vi "Main.vi"(10 "VISA resource name":refnum<visa-resource-name>, 11 "Module Admin":refnum<class "Delacor_lib_QMH_Cloneable Module Admin.lvclass">) -> ()   [LabVIEW 2018, in "CE14_v3.lvlib"]
doc: "This template is based off of the Queued Message Handler design pattern and the Queued Message Handler project template that ships with LabVIEW.\n\nThe main difference is that the queue is private to this module and communication between modules is performed via Broadcast and Request events.\n\nRequest events are wrapped in public API methods and are handled in the Event Handling Loop (EHL) of this VI. Any module can register for Broadcast events sent by this module. The EHL generates messages based on user interface actions.\n\nThe Message Handling Loop (MHL) processes messages generated by the EHL, or by other messages. The messages are string values, so new messages can be added easily to the Message Cases case structure in the MHL. Each message cluster can also provide an optional value for Message Data, which is a variant that can be converted to whatever message-specific data is required.\n_____\nBased on DQMH Project Template 6.0.0.91."
uses:
  CE14_v3.lvlib
  <vilib>/Delacor/Delacor QMH/Libraries/Cloneable Module Admin_class/Delacor_lib_QMH_Cloneable Module Admin.lvclass
  C:/Program Files (x86)/National Instruments/LabVIEW 2018/vi.lib/Delacor/Delacor QMH/Libraries/Module Admin_class/Delacor_lib_QMH_Module Admin.lvclass
  Module Data--cluster.ctl
  <vilib>/Delacor/Delacor QMH/Libraries/Message Queue_class/Delacor_lib_QMH_Message Queue.lvclass/Delacor_lib_QMH_Message Queue.ctl
  <vilib>/Delacor/Delacor QMH/Libraries/Cloneable Module Admin_class/Delacor_lib_QMH_Cloneable Module Admin.lvclass/Delacor_lib_QMH_Cloneable Module Admin.ctl
  Stop Argument--cluster.ctl
  <vilib>/Delacor/Delacor QMH/Libraries/Module Admin_class/Delacor_lib_QMH_Module Admin.lvclass/Delacor_lib_QMH_Module Admin.ctl
  CE14 Open and Shakehand Argument--cluster.ctl
  Check Shakehand Success Argument--cluster.ctl
  Check Shakehand Success (Reply Payload)--cluster.ctl
  <vilib>/Utility/miscctls.llb/LVPointTypeDef.ctl
  <vilib>/Delacor/Delacor QMH/Libraries/Message Queue_class/Delacor_lib_QMH_Enqueue Message (Single).vi
  <vilib>/Delacor/Delacor QMH/Libraries/Cloneable Module Admin_class/Delacor_lib_QMH_Get Module ID.vi
  <vilib>/Delacor/Delacor QMH/Libraries/Module Admin_class/Delacor_lib_QMH_Get External Launch.vi
  <vilib>/Utility/error.llb/Error Cluster From Error Code.vi
  <vilib>/ErrorRing/Error Ring.xnode
  <vilib>/Delacor/Delacor QMH/Libraries/Message Queue_class/Delacor_lib_QMH_Message Queue.lvclass
  Instrument Drivers/LVdriver_CE14(eMIC)/CE14_eMIC.lvlib
panel:
  out "error out":errorcluster
  out "Status":string
  in  "Simulate EHL Error":bool
  in  "Simulate MHL Error":bool
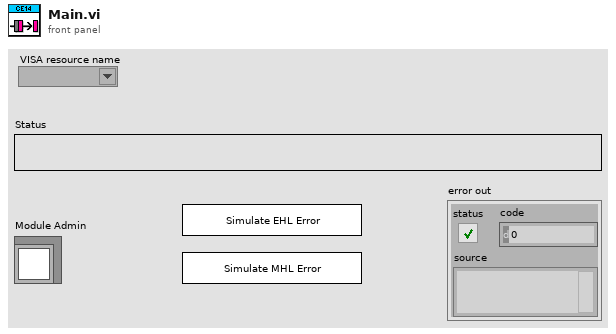
[diagram p1: front panel]
types:
  T1 = typedef "CE14_v3.lvlib/Request Events--cluster.ctl" = cluster{"Stop Module":refnum<user-event>, "Show Panel":refnum<user-event>, "Hide Panel":refnum<user-event>, "Show Diagram":refnum<user-event>, "Get Module Execution Status":refnum<user-event>, "CE14 Open and Shakehand":refnum<user-event>, "Check Shakehand Success":refnum<user-event>}
  T2 = typedef "CE14_v3.lvlib/Module Data--cluster.ctl" = cluster{"Status":string, "VISA resource name":refnum<visa-resource-name>, "ShakeHand Success?":bool}
  T3 = enum32{"invalid lock state", "Not Locked", "Locked (No Password)", "Password-protected"}
  T4 = typedef "CE14_v3.lvlib/Stop Argument--cluster.ctl" = cluster{"Module ID":i32, "Origin":string, "Exit via Stop Module Req?":bool, "Wait for Module to stop?":bool}
  T5 = typedef "CE14_v3.lvlib/CE14 Open and Shakehand Argument--cluster.ctl" = cluster{"Module ID":i32, "Boolean":bool}
  T6 = typedef "CE14_v3.lvlib/Check Shakehand Success Argument--cluster.ctl" = cluster{"Module ID":i32, "Wait Notifier":refnum<notifier>, "wait for reply":bool}
  T7 = typedef "LVPointTypeDef.ctl" = cluster{"Horizontal":i16, "Vertical":i16}
  T8 = enum32{"Invalid", "Standard", "Closed", "Hidden", "Minimized", "Maximized"}
  T9 = typedef "CE14_v3.lvlib/Check Shakehand Success (Reply Payload)--cluster.ctl" = cluster{"ShakeHand Success?":bool, "Check Shakehand Success_error":errorcluster}
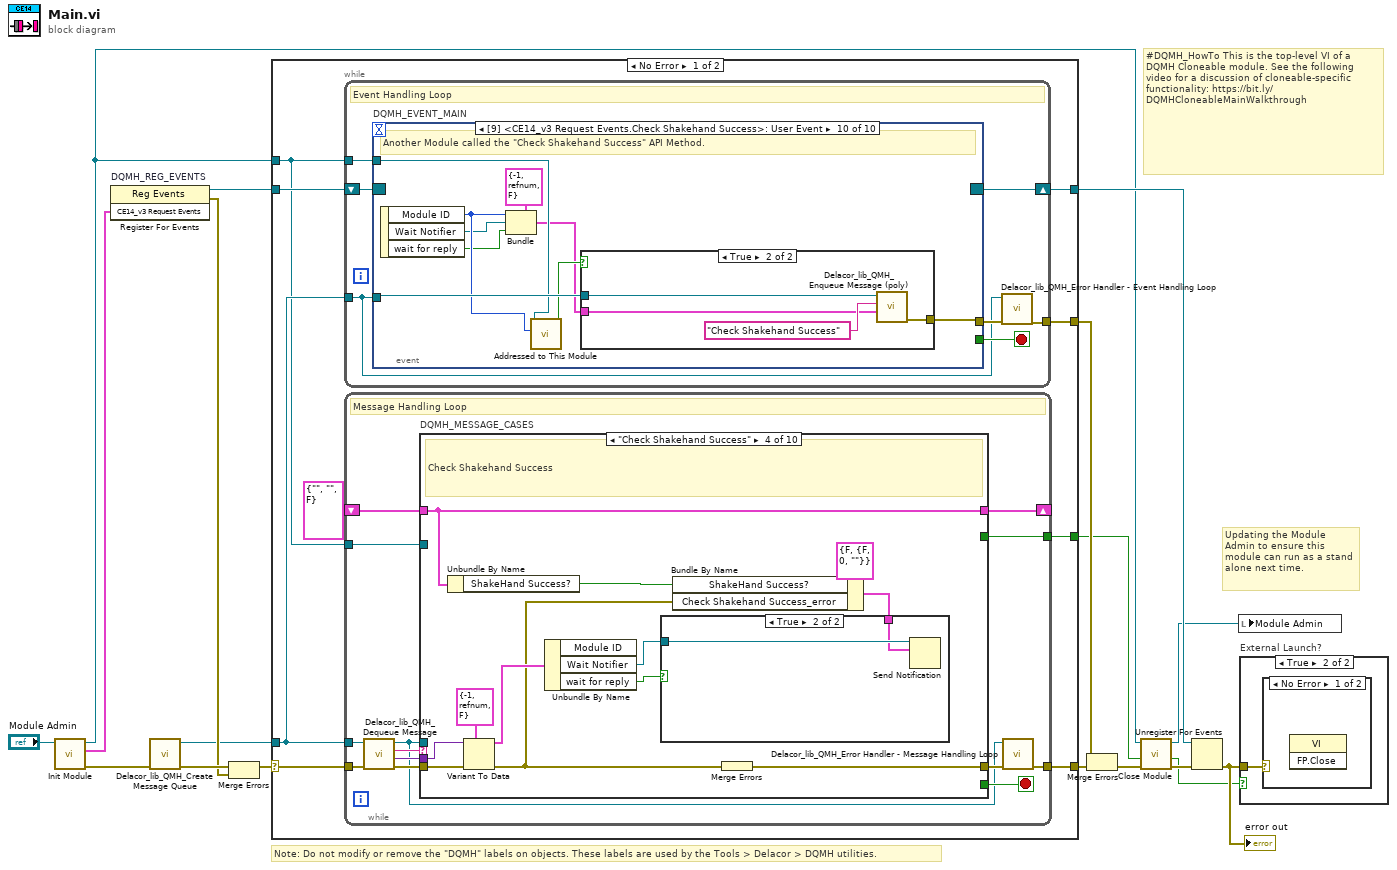
[diagram p0: block diagram]
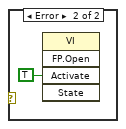
[diagram p3: hidden frame]
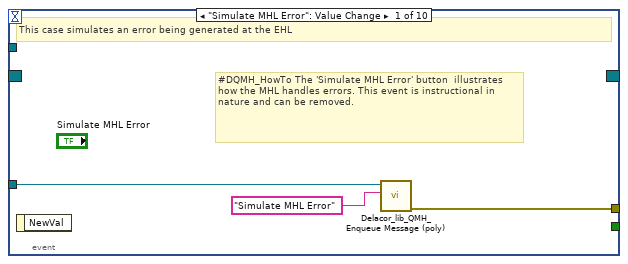
[diagram p4: hidden frame]
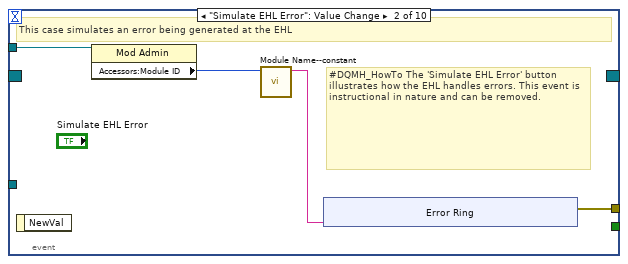
[diagram p5: hidden frame]
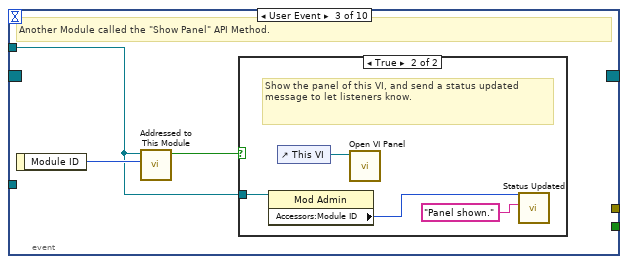
[diagram p6: hidden frame]
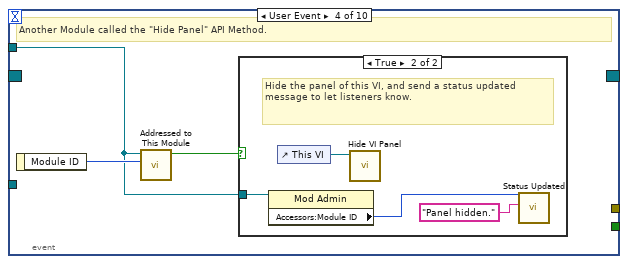
[diagram p8: hidden frame]
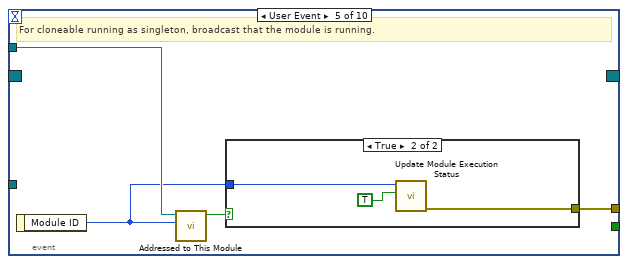
[diagram p10: hidden frame]
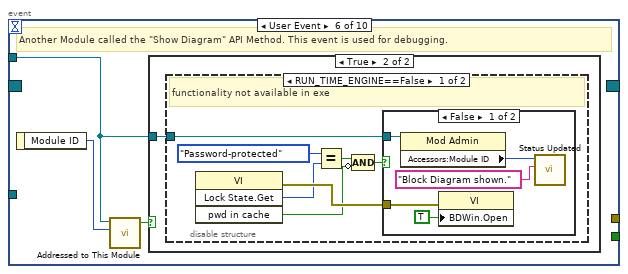
[diagram p12: hidden frame]
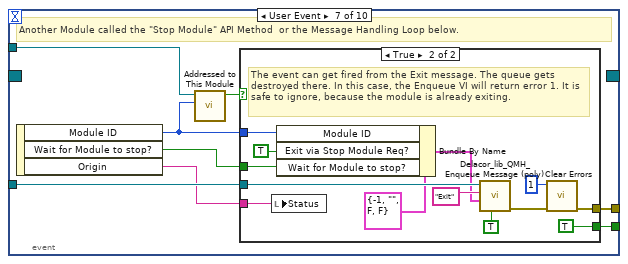
[diagram p16: hidden frame]
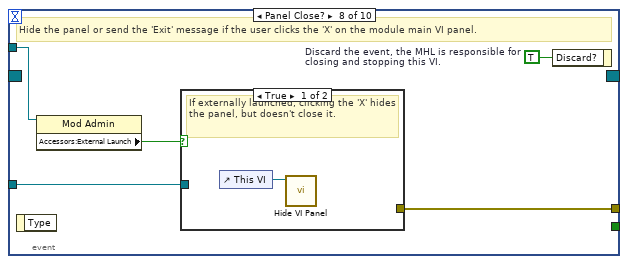
[diagram p18: hidden frame]
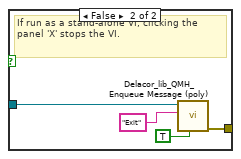
[diagram p19: hidden frame]
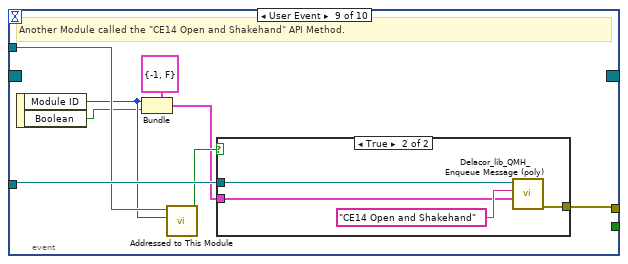
[diagram p20: hidden frame]
diagram:
  # "#DQMH_HowTo This is the top-level VI of a DQMH Cloneable module. See the following video for a discussion of cloneable-specific functionality: https://bit.ly/DQMHCloneableMainWalkthrough"
  # "Note: Do not modify or remove the \"DQMH\" labels on objects. These labels are used by the Tools > Delacor > DQMH utilities."
  # "Updating the Module Admin to ensure this module can run as a stand alone next time."
  n1 = call "Init Module.vi"("Cloneable Module Admin in"="Module Admin") -> ("error out"=w15:errorcluster, "CE14_v3 Request Events"=w7:T1, "Cloneable Module Admin out"=w4:refnum<class "Delacor_lib_QMH_Cloneable Module Admin.lvclass">)  [unwired: 8 in]
  n2 = register-events "DQMH_REG_EVENTS"(w7) -> (reference out=w8:refnum<event-registration>, error out=w10:errorcluster)  [unwired: 2 in]
  n3 = call <vilib>:"Delacor_lib_QMH_Create Message Queue.vi"("error in"=w15) -> ("error out"=w12:errorcluster, "Message Queue"=w6:refnum<class "Delacor_lib_QMH_Message Queue.lvclass">)  [unwired: 9 in]
  n4 = Merge Errors(w12, w10) -> (w11:errorcluster)
  n5 = case shown="No Error" w11 {
    selector: w11 -> [w25 w274]
    tunnel: [w27 w273] -> w16
    tunnel: [w24 w281] -> w9
    tunnel: w8 -> [w22 w281]
    tunnel: w6 -> [w21 w272]
    tunnel: [w26 _] -> w17
    tunnel: w4 -> [w20 w277]
    tunnel: [w19 _] -> w2
    frame No Error {
      n6 = while {
        tunnel: w21 -> [w28]
        shift-right: [w31] -> w24
        shift-left: w22 -> [w32]
        tunnel: [w33] -> w26
        tunnel: w20 -> [w29]
        stop <- w30 stop-if-true
        # "Event Handling Loop"
        n7 = event "DQMH_EVENT_MAIN" shown="[9] <CE14_v3 Request Events.Check Shakehand Success>: User Event" {
          selector: w32 -> [_ _ _ _ _ _ _ _ _ _]
          dyn-events: [_ _ _ _ _ _ _ _ _ _] -> w31
          timeout: _ -> [_ _ _ _ _ _ _ _ _ _]
          tunnel: [_ _ _ _ _ _ w89 _ _ _] -> w30
          tunnel: w28 -> [w36 _ _ _ _ _ w92 w108 w124 w137]
          tunnel: [w37 w41 _ _ w66 _ w93 w111 w117 w129] -> w34
          tunnel: w29 -> [_ w40 w49 w56 w64 w70 w91 w109 w122 w135]
          event "Simulate MHL Error": Value Change {
            # "#DQMH_HowTo The 'Simulate MHL Error' button  illustrates how the MHL handles errors. This event is instructional in nature and can be removed."
            # "This case simulates an error being generated at the EHL"
            n8 = event-data() -> ()  [unwired: 1 in, 1 out]
            n9 = call-poly <vilib>:"Delacor_lib_QMH_Enqueue Message (poly).vi"("Message"="Simulate MHL Error", "Message Queue in"=w36) -> ("error out"=w37:errorcluster)  [unwired: 8 in, 1 out]
          }
          event "Simulate EHL Error": Value Change {
            # "#DQMH_HowTo The 'Simulate EHL Error' button  illustrates how the EHL handles errors. This event is instructional in nature and can be removed."
            # "This case simulates an error being generated at the EHL"
            n10 = event-data() -> ()  [unwired: 1 in, 1 out]
            n11 = property class="Mod Admin"(reference=w40) -> ("Accessors:Module ID"=w39:i32)  [unwired: 1 in, 2 out]
            n12 = call "Module Name--constant.vi"("Module ID"=w39) -> ("Module Name"=w38:string)  [unwired: 10 in]
            n13 = xnode "Error Ring"("parameter 0"=w38) -> ("error out"=w41:errorcluster)
          }
          event User Event {
            # "Another Module called the \"Show Panel\" API Method."
            n14 = event-data() -> ("Module ID"=w50:i32)  [unwired: 1 in]
            n15 = call "Addressed to This Module.vi"("Module ID from Argument"=w50, "Module Admin"=w49) -> ("Addressed to this instance?"=w51:bool)  [unwired: 8 in, 1 out]
            n16 = case shown="True" w51 {
              tunnel: w49 -> [_ w53]
              frame False {
              }
              frame True {
                # "Show the panel of this VI, and send a status updated message to let listeners know."
                n17 = property class="Mod Admin"(reference=w53) -> ("Accessors:Module ID"=w52:i32)  [unwired: 1 in, 2 out]
                n18 = control-ref of="This VI"() -> (w55:refnum<vi>)
                n19 = call "Open VI Panel.vi"("VI"=w55) -> ()  [unwired: 10 in, 1 out]
                n20 = call "Status Updated.vi"("Status"="Panel shown." ("format string"), "Module ID"=w52) -> ()  [unwired: 9 in, 1 out]
              }
            }
          }
          event User Event {
            # "Another Module called the \"Hide Panel\" API Method."
            n21 = event-data() -> ("Module ID"=w57:i32)  [unwired: 1 in]
            n22 = call "Addressed to This Module.vi"("Module ID from Argument"=w57, "Module Admin"=w56) -> ("Addressed to this instance?"=w58:bool)  [unwired: 8 in, 1 out]
            n23 = case shown="True" w58 {
              tunnel: w56 -> [_ w60]
              frame False {
              }
              frame True {
                # "Hide the panel of this VI, and send a status updated message to let listeners know."
                n24 = property class="Mod Admin"(reference=w60) -> ("Accessors:Module ID"=w59:i32)  [unwired: 1 in, 2 out]
                n25 = control-ref of="This VI"() -> (w62:refnum<vi>)
                n26 = call "Hide VI Panel.vi"("VI"=w62) -> ()  [unwired: 10 in, 1 out]
                n27 = call "Status Updated.vi"("Status"="Panel hidden." ("format string"), "Module ID"=w59) -> ()  [unwired: 9 in, 1 out]
              }
            }
          }
          event User Event {
            # "For cloneable running as singleton, broadcast that the module is running."
            n28 = event-data() -> ("Module ID"=w63:i32)  [unwired: 1 in]
            n29 = call "Addressed to This Module.vi"("Module ID from Argument"=w63, "Module Admin"=w64) -> ("Addressed to this instance?"=w65:bool)  [unwired: 8 in, 1 out]
            n30 = case shown="True" w65 {
              tunnel: [_ w69] -> w66
              tunnel: w63 -> [_ w68]
              frame False {
              }
              frame True {
                n31 = call "Update Module Execution Status.vi"("Running?"=TRUE, "Module ID"=w68) -> ("error out"=w69:errorcluster)  [unwired: 9 in]
              }
            }
          }
          event User Event {
            # "Another Module called the \"Show Diagram\" API Method. This event is used for debugging."
            n32 = event-data() -> ("Module ID"=w71:i32)  [unwired: 1 in]
            n33 = call "Addressed to This Module.vi"("Module ID from Argument"=w71, "Module Admin"=w70) -> ("Addressed to this instance?"=w72:bool)  [unwired: 8 in, 1 out]
            n34 = case shown="True" w72 {
              tunnel: w70 -> [_ w73]
              frame False {
              }
              frame True {
                n35 = disable-structure shown="RUN_TIME_ENGINE==False" {
                  disable-tunnel: w73 -> [w74 _]
                  frame condition #0 (active) {
                    # "functionality not available in exe"
                    n36 = invoke class="VI" method="Lock State.Get"() -> (error out=w80:errorcluster, "Get Lock State"=w79:T3, "pwd in cache"=w76:bool)  [unwired: 4 in, 1 out]
                    n37 = Equal?(x=T3."Password-protected", y=w79) -> (x = y?=w77:bool)
                    n38 = Compound Arithmetic op=AND(w77, invert w76) -> (w75:bool)
                    n39 = case shown="False" w75 {
                      tunnel: w80 -> [w85 _]
                      tunnel: w74 -> [w82 _]
                      frame False {
                        n40 = property class="Mod Admin"(reference=w82) -> ("Accessors:Module ID"=w81:i32)  [unwired: 1 in, 2 out]
                        n41 = property class="VI"(error in=w85, "BDWin.Open"=TRUE ("Block Diagram Window:Open")) -> ()  [unwired: 1 in, 2 out]
                        n42 = call "Status Updated.vi"("Status"="Block Diagram shown." ("format string"), "Module ID"=w81) -> ()  [unwired: 9 in, 1 out]
                      }
                      frame True {
                        # "Password-protected VI, and the password is not in the cache. Do not show the diagram."
                      }
                    }
                  }
                  frame condition #1 {
                  }
                }
              }
            }
          }
          event User Event {
            # "Another Module called the \"Stop Module\" API Method  or the Message Handling Loop below."
            n43 = event-data() -> ("Module ID"=w87:i32, "Wait for Module to stop?"=w88:bool, "Origin"=w86:string)  [unwired: 1 in]
            n44 = call "Addressed to This Module.vi"("Module ID from Argument"=w87, "Module Admin"=w91) -> ("Addressed to this instance?"=w90:bool)  [unwired: 8 in, 1 out]
            n45 = case shown="True" w90 {
              tunnel: [_ w105] -> w93
              tunnel: w92 -> [_ w101]
              tunnel: [_ TRUE] -> w89
              tunnel: w88 -> [_ w96]
              tunnel: w87 -> [_ w98]
              tunnel: w86 -> [_ w94]
              frame False {
              }
              frame True {
                # "The event can get fired from the Exit message. The queue gets destroyed there. In this case, the Enqueue VI will return error 1. It is safe to ignore, because the module is already exiting."
                n46 = local write "Status"(w94) -> ()
                n47 = Bundle By Name(cluster=T4 {"Module ID"=-1, "Origin"="", "Exit via Stop Module Req?"=FALSE, "Wait for Module to stop?"=FALSE} ("Stop Argument"), "Module ID"=w98, "Exit via Stop Module Req?"=TRUE, "Wait for Module to stop?"=w96) -> (w95:T4)
                n48 = call-poly <vilib>:"Delacor_lib_QMH_Enqueue Message (poly).vi"("Priority Message? (F)"=TRUE, "Message Data"=w95, "Message"="Exit", "Message Queue in"=w101) -> ("error out"=w106:errorcluster)  [unwired: 6 in, 1 out]
                n49 = call <vilib>:"Clear Errors.vi"("error in (no error)"=w106, "specific error code to clear (0: all)"=1) -> ("error out"=w105:errorcluster)  [unwired: 4 in, 1 out]
              }
            }
          }
          event Panel Close? {
            w110 = TRUE  # Discard the event, the MHL is responsible for closing and stopping this VI.
            # "Hide the panel or send the 'Exit' message if the user clicks the 'X' on the module main VI panel."
            n50 = event-data() -> ()  [unwired: 1 in, 1 out]
            n51 = property class="Mod Admin"(reference=w109) -> ("Accessors:External Launch"=w107:bool)  [unwired: 1 in, 2 out]
            n52 = case shown="True" w107 {
              tunnel: w108 -> [_ w115]
              tunnel: [_ w116] -> w111
              frame True {
                # "If externally launched, clicking the 'X' hides the panel, but doesn't close it."
                n53 = control-ref of="This VI"() -> (w112:refnum<vi>)
                n54 = call "Hide VI Panel.vi"("VI"=w112) -> ()  [unwired: 10 in, 1 out]
              }
              frame False {
                # "If run as a stand-alone VI, clicking the panel 'X' stops the VI."
                n55 = call-poly <vilib>:"Delacor_lib_QMH_Enqueue Message (poly).vi"("Priority Message? (F)"=TRUE, "Message"="Exit", "Message Queue in"=w115) -> ("error out"=w116:errorcluster)  [unwired: 7 in, 1 out]
              }
            }
            n56 = event-data("Discard?"=w110) -> ()  [unwired: 1 in, 1 out]
          }
          event User Event {
            # "Another Module called the \"CE14 Open and Shakehand\" API Method."
            n57 = event-data() -> ("Module ID"=w119:i32, "Boolean"=w118:bool)  [unwired: 1 in]
            n58 = Bundle(cluster=T5 {"Module ID"=-1, "Boolean"=FALSE} ("CE14 Open and Shakehand Argument"), "Module ID"=w119, "Boolean"=w118) -> (w120:T5)
            n59 = call "Addressed to This Module.vi"("Module ID from Argument"=w119, "Module Admin"=w122) -> ("Addressed to this instance?"=w123:bool)  [unwired: 8 in, 1 out]
            n60 = case shown="True" w123 {
              tunnel: w124 -> [_ w128]
              tunnel: w120 -> [_ w126]
              tunnel: [_ w125] -> w117
              frame False {
              }
              frame True {
                n61 = call-poly <vilib>:"Delacor_lib_QMH_Enqueue Message (poly).vi"("Message Data"=w126, "Message"="CE14 Open and Shakehand", "Message Queue in"=w128) -> ("error out"=w125:errorcluster)  [unwired: 7 in, 1 out]
              }
            }
          }
          event User Event {
            # "Another Module called the \"Check Shakehand Success\" API Method."
            n62 = event-data() -> ("Module ID"=w132:i32, "Wait Notifier"=w131:refnum<notifier>, "wait for reply"=w130:bool)  [unwired: 1 in]
            n63 = Bundle(cluster=T6 {"Module ID"=-1, "Wait Notifier"=refnum, "wait for reply"=FALSE} ("Check Shakehand Success Argument"), "Module ID"=w132, "Wait Notifier"=w131, "wait for reply"=w130) -> (w133:T6)
            n64 = call "Addressed to This Module.vi"("Module ID from Argument"=w132, "Module Admin"=w135) -> ("Addressed to this instance?"=w136:bool)  [unwired: 8 in, 1 out]
            n65 = case shown="True" w136 {
              tunnel: w137 -> [_ w141]
              tunnel: w133 -> [_ w139]
              tunnel: [_ w138] -> w129
              frame False {
              }
              frame True {
                n66 = call-poly <vilib>:"Delacor_lib_QMH_Enqueue Message (poly).vi"("Message Data"=w139, "Message"="Check Shakehand Success", "Message Queue in"=w141) -> ("error out"=w138:errorcluster)  [unwired: 7 in, 1 out]
              }
            }
          }
        }
        n67 = call-dynamic "Delacor_lib_QMH_Error Handler - Event Handling Loop.vi"("error in"=w34, "Message Queue in"=w28) -> ("dup error in"=w33:errorcluster)  [unwired: 8 in, 1 out]
      }
      n68 = while {
        tunnel: w21 -> [w145]
        shift-right: [w149] -> _
        shift-left: T2 {"Status"="", "VISA resource name"="", "ShakeHand Success?"=FALSE} ("Data Cluster") -> [w150]
        tunnel: w25 -> [w153]
        tunnel: [w151] -> w27
        tunnel: w20 -> [w143]
        tunnel: [w142] -> w19
        stop <- w148 stop-if-true
        # "Message Handling Loop"
        n69 = call-dynamic "Delacor_lib_QMH_Dequeue Message.vi"("error in"=w153, "Message Queue in"=w145) -> ("error out"=w152:errorcluster, "Message Data"=w146:variant, "Message"=w147:string, "Message Queue out"=w144:refnum<class "Delacor_lib_QMH_Message Queue.lvclass">)  [unwired: 6 in]
        n70 = case "DQMH_MESSAGE_CASES" shown="\"Check Shakehand Success\"" w147 {
          selector: w147 -> [_ _ _ _ _ _ _ _ _ w259]
          tunnel: w144 -> [_ _ _ _ _ _ w210 _ w249 _]
          tunnel: w152 -> [w175 w179 w189 w201 w206 w208 w219 w232 w255 w261]
          tunnel: [w173 w179 w183 w193 w205 w208 w215 w231 w252 w262] -> w154
          tunnel: w150 -> [w155 w178 w180 w192 w204 w207 w214 w229 w248 w260]
          tunnel: [w166 w178 w181 w192 w204 w207 w214 w229 w248 w260] -> w149
          tunnel: [_ _ _ _ _ _ _ _ w247 _] -> w148
          tunnel: w146 -> [_ _ w188 w200 _ _ w213 _ w245 _]
          tunnel: w143 -> [w161 _ _ _ _ _ w212 w227 w241 w257]
          tunnel: [_ _ _ _ _ _ _ _ w243 _] -> w142
          frame "Initialize" {
            w158 = "Initial Message" ("Initial Message")
            # "Initialize - Any operation that needs to be done before the module can receive messages. Synchronize Caller Events.vi will inform Start Module.vi that the module has launched and is ready to receive messages. Module Did Init.vi will broadcast that the module initialized."
            n71 = call "Synchronize Caller Events.vi"("error in (no error)"=w175, "Module Admin"=w161) -> ("error out"=w174:errorcluster, "Module Admin out"=w160:refnum<class "Delacor_lib_QMH_Cloneable Module Admin.lvclass">)  [unwired: 8 in]
            n72 = property class="Mod Admin"(reference=w160) -> ("Accessors:Module ID"=w163:i32, "Accessors:External Launch"=w162:bool)  [unwired: 1 in, 2 out]
            n73 = Bundle By Name(cluster=w155, "VISA resource name"="VISA resource name") -> (w156:T2)
            n74 = call "Module Name--constant.vi"("Module ID"=w163) -> ("Module Name"=w170:string)  [unwired: 10 in]
            n75 = property class="VI"("Front Panel.Title"=w170) -> (reference out=w172:refnum<vi>, error out=w177:errorcluster)  [unwired: 2 in]
            n76 = Select(t=T8."Hidden" ("State"), s=w162, f=T8."Standard" ("State")) -> (s? t:f=w167:T8)
            n77 = invoke class="VI" method="FP.Open"(reference=w172, error in=w177, "State"=w167) -> (reference out=w171:refnum<vi>, error out=w176:errorcluster)  [unwired: 2 in, 3 out]
            n78 = call "Module Name--constant.vi"("Module ID"=w163) -> ("Module Name"=w164:string)  [unwired: 10 in]
            n79 = Bundle By Name(cluster=w156, "Status"=w158) -> (w166:T2)
            n80 = invoke class="VI" method="FP.Center"(reference=w171, error in=w176) -> ()  [unwired: 1 in, 3 out]
            n81 = property on="Pane" class="Pane"("Origin"=T7 {"Horizontal"=0, "Vertical"=0}) -> ()  [unwired: 2 in, 2 out]
            n82 = call "Module Did Init.vi"("error in (no error)"=w174, "Initialized?"=TRUE, "Origin"=w164, "Module ID"=w163) -> ("error out"=w173:errorcluster)  [unwired: 7 in]
            "Status" <- w158
          }
          frame "---Module Specific---" {
            # "Separator -- The following cases handle messages specific to this Module."
          }
          frame "CE14 Open and Shakehand" {
            # "Open and Shakehand eMIC CE14"
            n83 = Unbundle By Name(w180) -> ("VISA resource name"=w186:refnum<visa-resource-name>)
            n84 = Variant To Data(error in=w189, type=T5 {"Module ID"=-1, "Boolean"=FALSE} ("CE14 Open and Shakehand Argument"), Variant=w188) -> (error out=w184:errorcluster)  [unwired: 1 out]
            n85 = call "CE14.open handshake(subVI).vi"("VISA resource name"=w186) -> ("error out"=w182:errorcluster, "success"=w185:bool)  [unwired: 7 in, 2 out]
            n86 = Bundle By Name(cluster=w180, "ShakeHand Success?"=w185) -> (w181:T2)
            n87 = Merge Errors(w184, w182) -> (w183:errorcluster)
          }
          frame "Check Shakehand Success" {
            # "Check Shakehand Success"
            n88 = Unbundle By Name(w192) -> ("ShakeHand Success?"=w191:bool)
            n89 = Variant To Data(error in=w201, type=T6 {"Module ID"=-1, "Wait Notifier"=refnum, "wait for reply"=FALSE} ("Check Shakehand Success Argument"), Variant=w200) -> (data=w198:T6, error out=w190:errorcluster)
            n90 = Unbundle By Name(w198) -> ("Wait Notifier"=w197:refnum<notifier>, "wait for reply"=w196:bool)  [unwired: 1 out]
            n91 = Bundle By Name(cluster=T9 {"ShakeHand Success?"=FALSE, "Check Shakehand Success_error"={"status"=FALSE, "code"=0, "source"=""}} ("Check Shakehand Success (Reply Payload)"), "ShakeHand Success?"=w191, "Check Shakehand Success_error"=w190) -> (w195:T9)
            n92 = case shown="True" w196 {
              tunnel: w197 -> [_ w203]
              tunnel: w195 -> [_ w202]
              frame False {
              }
              frame True {
                n93 = Send Notification(notification=w202, notifier=w203) -> ()  [unwired: 1 in, 2 out]
              }
            }
            n94 = Merge Errors(w190) -> (w193:errorcluster)
          }
          frame "---Copy This Frame---" {
            # "Duplicate this frame when creating new messages.  Change this comment in the duplicated frame to describe this message."
            n95 = Merge Errors(w206) -> (w205:errorcluster)
          }
          frame "---Exit and Error Handling---" {
            # "Separator - the following cases handle errors and exit messages."
          }
          frame "Error" {
            # "#CodeRecommended - If you ever change the name of this \"Error\" message, you'll need to update the name in the Check Loop Error.vi as well."
            # "#CodeRecommended - If the module is running in standalone mode (External Launch = FALSE), this code will pop up an error dialog and call the 'Exit' message if an error occurs. Add more fine-grained error handling here."
            # "Error - Check the error message data and respond accordingly. This message is sent by the \"Error Handler\" VIs at the end of each loop in this application."
            n96 = property class="Mod Admin"(reference=w212) -> ("Accessors:External Launch"=w211:bool, "Accessors:Module ID"=w209:i32)  [unwired: 1 in, 2 out]
            n97 = Variant To Data(error in=w219, type=errorcluster {"status"=FALSE, "code"=0, "source"=""} ("error constant"), Variant=w213) -> (data=w220:errorcluster, error out=w217:errorcluster)
            n98 = call "Error Reported.vi"("Error"=w220, "Module ID"=w209) -> ()  [unwired: 9 in, 1 out]
            n99 = case shown="False" w211 {
              tunnel: [w225 _] -> w216
              tunnel: w210 -> [w223 _]
              tunnel: w220 -> [w224 _]
              frame False {
                # "If the module is running standalone, then pop up an error dialog and call the \"Exit\" message."
                n100 = call <vilib>:"Simple Error Handler.vi"("error in (no error)"=w224) -> ()  [unwired: 4 in, 5 out]
                n101 = call-poly <vilib>:"Delacor_lib_QMH_Enqueue Message (poly).vi"("Priority Message? (F)"=TRUE, "Message"="Exit", "Message Queue in"=w223) -> ("error out"=w225:errorcluster)  [unwired: 7 in, 1 out]
              }
              frame True {
                # "If the module was launched externally, calling the Error Reported broadcast VI is the only action performed by the \"Error\" message. The module's caller can then process the error appropriately."
              }
            }
            n102 = Merge Errors(w217, w216) -> (w215:errorcluster)
            n103 = local write "error out"(w215) -> ()
          }
          frame "Simulate MHL Error" {
            # "#DQMH_HowTo The 'Simulate MHL Error' button  illustrates how the MHL handles errors. This event is instructional in nature and can be removed."
            # "Simulate an error occurring at the MHL"
            n104 = property class="Mod Admin"(reference=w227) -> ("Accessors:Module ID"=w228:i32)  [unwired: 1 in, 2 out]
            n105 = call "Module Name--constant.vi"("Module ID"=w228) -> ("Module Name"=w226:string)  [unwired: 10 in]
            n106 = xnode "Error Ring"("parameter 0"=w226) -> ("error out"=w230:errorcluster)
            n107 = Merge Errors(w232, w230) -> (w231:errorcluster)
          }
          frame "Exit" {
            w246 = 91  # 91: not all Exit messages will have an argument
            w247 = TRUE  # Stop the VI
            # "Release the message queue reference"
            # "#CodeNeeded - Add any required cleanup code here."
            # "Exit - Exit the application."
            n108 = Variant To Data(error in=w255, type=T4 {"Module ID"=-1, "Origin"="", "Exit via Stop Module Req?"=FALSE, "Wait for Module to stop?"=FALSE} ("Stop Argument"), Variant=w245) -> (data=w242:T4, error out=w250:errorcluster)
            n109 = call <vilib>:"Clear Errors.vi"("error in (no error)"=w250, "specific error code to clear (0: all)"=w246) -> ("error out"=w254:errorcluster)  [unwired: 4 in, 1 out]
            n110 = control-ref of="This VI"() -> (w240:refnum<vi>)
            n111 = call-dynamic "Delacor_lib_QMH_Release Message Queue.vi"("error in"=w254, "Message Queue"=w249) -> ("error out"=w253:errorcluster)  [unwired: 9 in]
            n112 = call "Handle Exit.vi"("Stop Argument"=w242, "Module Admin in"=w241, "VI reference"=w240) -> ("error out"=w251:errorcluster, "Wait for Stop?"=w243:bool)  [unwired: 7 in]
            n113 = Merge Errors(w253, w251) -> (w252:errorcluster)
          }
          frame Default {
            # "'Default' case only runs if there is a message that isn't defined in any of the other cases.  Output a programming error."
            n114 = property class="Mod Admin"(reference=w257) -> ("Accessors:Module ID"=w256:i32)  [unwired: 1 in, 2 out]
            n115 = call "Module Name--constant.vi"("Module ID"=w256) -> ("Module Name"=w258:string)  [unwired: 10 in]
            n116 = xnode "Error Ring"("parameter 0"=w259, "parameter 1"=w258) -> ("error out"=w263:errorcluster)
            n117 = Merge Errors(w261, w263) -> (w262:errorcluster)
          }
        }
        n118 = call-dynamic "Delacor_lib_QMH_Error Handler - Message Handling Loop.vi"("error in"=w154, "Message Queue in"=w144) -> ("dup error in"=w151:errorcluster)  [unwired: 8 in, 1 out]
      }
    }
    frame Error {
      n119 = call "Synchronize Caller Events.vi"("Module Admin"=w277) -> ("Module Admin out"=w276:refnum<class "Delacor_lib_QMH_Cloneable Module Admin.lvclass">)  [unwired: 9 in, 1 out]
      n120 = property class="Mod Admin"(reference=w276) -> ("Accessors:Module ID"=w275:i32)  [unwired: 1 in, 2 out]
      n121 = call-dynamic "Delacor_lib_QMH_Release Message Queue.vi"("error in"=w274, "Message Queue"=w272) -> ("error out"=w273:errorcluster)  [unwired: 9 in]
      n122 = call "Module Name--constant.vi"("Module ID"=w275) -> ("Module Name"=w280:string)  [unwired: 10 in]
      n123 = Format Into String(format string="An error occurred during initialization. %s is no longer running.", w280) -> (resulting string=w278:string)  [unwired: 2 in, 1 out]
      n124 = call "Error Reported.vi"("Additional Information"=w278, "Error"=w273, "Module ID"=w275) -> ()  [unwired: 8 in, 1 out]
    }
  }
  n125 = Merge Errors(w17, w16) -> (w18:errorcluster)
  n126 = call "Close Module.vi"("error in"=w18, "Wait for stop?"=w2, "Module Admin in"=w4) -> ("error out"=w14:errorcluster, "External Launch"=w1:bool, "Module Admin out"=w3:refnum<class "Delacor_lib_QMH_Cloneable Module Admin.lvclass">)  [unwired: 6 in]
  n127 = Unregister For Events(event registration refnum=w9, error in=w14) -> (error out=w13:errorcluster)
  "error out" <- w13
  n128 = local write "Module Admin"(w3) -> ()
  n129 = case "External Launch?" shown="True" w1 {
    tunnel: w13 -> [_ w282]
    frame False {
    }
    frame True {
      n130 = case shown="No Error" w282 {
        frame No Error {
          n131 = invoke class="VI" method="FP.Close"() -> ()  [unwired: 3 in, 3 out]
        }
        frame Error {
          n132 = invoke class="VI" method="FP.Open"("Activate"=TRUE ("Activate?")) -> ()  [unwired: 4 in, 5 out]
        }
      }
    }
  }
